vi "hpanel_DO_disconnect_from_hydraharp.vi"(8 "error in (no error)":errorcluster, 11 "hydraharp_panel in":refnum<class "hydraharp_panel.lvclass">) -> (0 "error out":errorcluster, 3 "hydraharp_panel out":refnum<class "hydraharp_panel.lvclass">)   [LabVIEW 2015, in "hydraharp_panel.lvclass"]
uses:
  hydraharp_panel.lvclass
  hydraharp/hydraharp.lvclass
  UI/panel_class/panel.lvclass
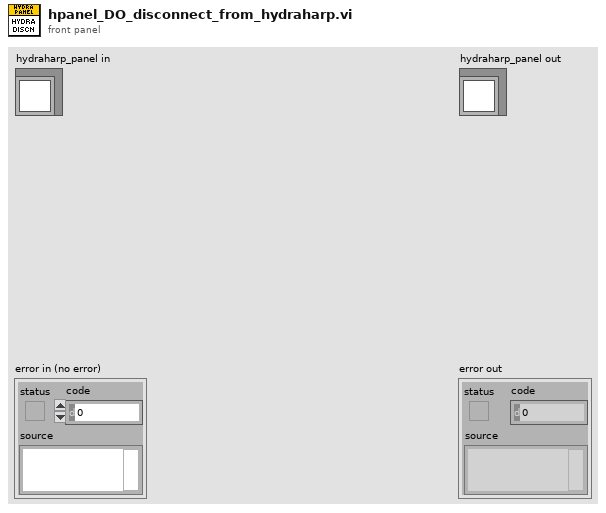
[diagram p1: front panel]
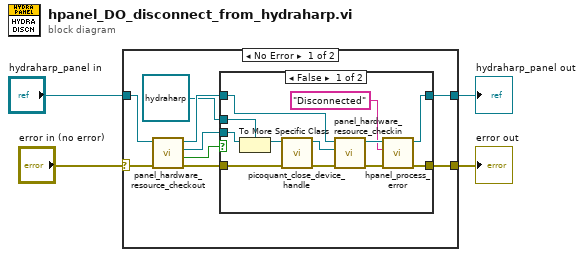
[diagram p0: block diagram]
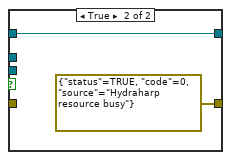
[diagram p2: hidden frame]
diagram:
  n1 = case shown="No Error" "error in (no error)" {
    selector: "error in (no error)" -> [w12 w29]
    tunnel: [w9 w29] -> w3
    tunnel: [w5 w28] -> w1
    tunnel: "hydraharp_panel in" -> [w13 w28]
    frame No Error {
      n2 = call "panel_hardware_resource_checkout.vi"("error in (no error)"=w12, "panel in"=w13) -> ("error out"=w10:errorcluster, "timed out?"=w11:bool, "hardware.lvclass"=w7:refnum<class "hardware.lvclass">, "panel out"=w8:refnum<class "hydraharp_panel.lvclass">)  [unwired: 6 in]
      n3 = case shown="False" w11 {
        tunnel: w10 -> [w17 _]
        tunnel: [w19 errorcluster {"status"=TRUE, "code"=0, "source"="Hydraharp resource busy"} ("error out")] -> w9
        tunnel: w8 -> [w25 w26]
        tunnel: w7 -> [w23 _]
        tunnel: refnum<class "hydraharp.lvclass"> refnum ("hydraharp.lvclass") -> [w24 _]
        tunnel: [w18 w26] -> w5
        frame False {
          n4 = To More Specific Class(target class=w24, reference=w23) -> (specific class reference=w15:refnum<class "hydraharp.lvclass">)  [unwired: 1 in, 1 out]
          n5 = call-dynamic "picoquant_close_device_handle.vi"("error in (no error)"=w17, "hydraharp in"=w15) -> ("error out"=w16:errorcluster, "hydraharp out"=w14:refnum<class "hydraharp.lvclass">)  [unwired: 8 in]
          n6 = call "panel_hardware_resource_checkin.vi"("error in (no error)"=w16, "hardware.lvclass"=w14, "panel in"=w25) -> ("error out"=w22:errorcluster, "panel out"=w21:refnum<class "hydraharp_panel.lvclass">)  [unwired: 7 in]
          n7 = call "hpanel_process_error.vi"("error in (no error)"=w22, "No Error Message"="Disconnected" ("String"), "hydraharp_panel in"=w21) -> ("error out"=w19:errorcluster, "hydraharp_panel out"=w18:refnum<class "hydraharp_panel.lvclass">)  [unwired: 7 in]
        }
        frame True {
        }
      }
    }
    frame Error {
    }
  }
  "error out" <- w3
  "hydraharp_panel out" <- w1
